vi "createOutboundChannel.vi"(8 "error in (no error)":errorcluster, 10 "redirect":string, 11 "Connection.TCP in":refnum<class "Connection.TCP.lvclass">) -> (0 "error out":errorcluster, 3 "Connection.TCP out":refnum<class "Connection.TCP.lvclass">)   [LabVIEW 2013, in "Connection.TCP_GOSPL.lvlib" / "Connection.TCP.lvclass"]
uses:
  Connection.TCP.lvclass
  Connection/Connection.lvclass
  Connection/Connection.lvclass/Connection.ctl
  Connection.TCP.lvclass/Connection.TCP.ctl
  <vilib>/LabVIEW Open Source Project/OpenURI/openURI.lvlib
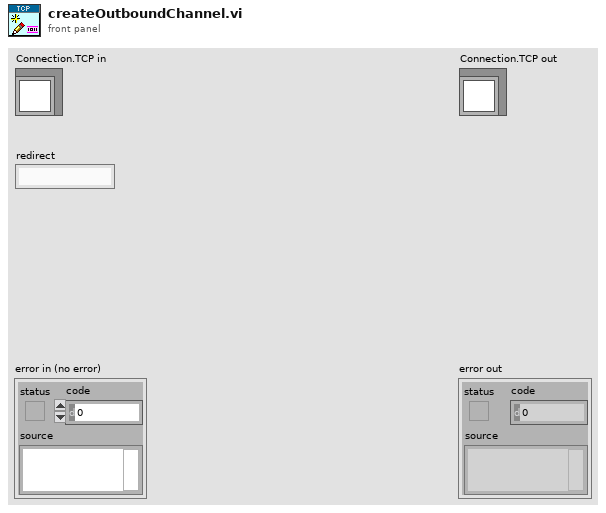
[diagram p1: front panel]
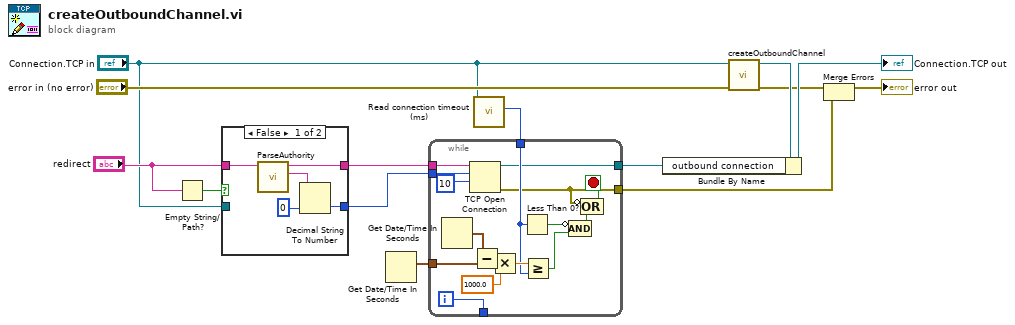
[diagram p0: block diagram]
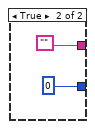
[diagram p2: hidden frame]
diagram:
  n1 = Empty String/Path?(string/path="redirect") -> (empty?=w2:bool)
  n2 = case shown="False" w2 {
    tunnel: [w17 u16 0 ("port")] -> w6
    tunnel: [w16 ""] -> w5
    tunnel: "redirect" -> [w15 _]
    tunnel: "Connection.TCP in" -> [_ _]
    frame False {
      n3 = call <vilib>:"ParseAuthority.vi"("authority"=w15) -> ("port"=w19:string, "host"=w16:string)  [unwired: 7 in, 2 out]
      n4 = Decimal String To Number(string=w19, default (0L)=u16 0 ("port")) -> (number=w17:u16)  [unwired: 1 in, 1 out]
    }
    frame True {
    }
  }
  n5 = Get Date/Time In Seconds() -> (seconds since 1Jan1904=w7:timestamp)
  n6 = call "Read connection timeout (ms).vi"("Connection in"="Connection.TCP in") -> ("connection timeout (ms)"=w4:i32)  [unwired: 8 in, 2 out]
  n7 = while {
    tunnel: [w26] -> w9
    tunnel: w4 -> [w29]
    tunnel: w7 -> [w37]
    tunnel: w6 -> [w28]
    tunnel: w5 -> [w24]
    tunnel: [w23] -> w8
    tunnel: [w22] -> _
    i -> [w22]
    stop <- w25 stop-if-true
    n8 = Get Date/Time In Seconds() -> (seconds since 1Jan1904=w36:timestamp)
    n9 = TCP Open Connection(address=w24, remote port or service name=w28, timeout ms (60000)=10 ("timeout in ms (-1)")) -> (connection ID=w26:refnum<k5>, error out=w23:errorcluster)  [unwired: 2 in]
    n10 = Subtract(x=w36, y=w37) -> (x-y=w35:dbl)
    n11 = Multiply(x=w35, y=1000.0) -> (x*y=w33:dbl)
    n12 = Less Than 0?(x=w29) -> (x < 0?=w30:bool)
    n13 = Greater Or Equal?(x=w33, y=w29) -> (x >= y?=w32:bool)
    n14 = Compound Arithmetic op=AND(invert w30, w32) -> (w31:bool)
    n15 = Compound Arithmetic op=OR(invert w23, w31) -> (w25:bool)
  }
  n16 = call-parent "createOutboundChannel.vi"("error in (no error)"="error in (no error)", "Connection in"="Connection.TCP in") -> ("error out"=w11:errorcluster, "Connection out"=w13:refnum<class "Connection.TCP.lvclass">)  [unwired: 8 in]
  n17 = Bundle By Name(cluster=w13, "outbound connection"=w9) -> (→"Connection.TCP out":refnum<class "Connection.TCP.lvclass">)
  n18 = Merge Errors(w11, w8) -> (→"error out":errorcluster)
